vi "identify objects.vi"(0 "location":cluster{"x":i16, "y":i16}, 1 "8-bit pixmap":u8[][](array[numeric]), 3 "index":u8, 4 "navigational matrix":T1(array[cluster])) -> (5 "direction":dbl[](array[numeric]), 6 "distance":u16[](array[numeric]))   [LabVIEW 2009]
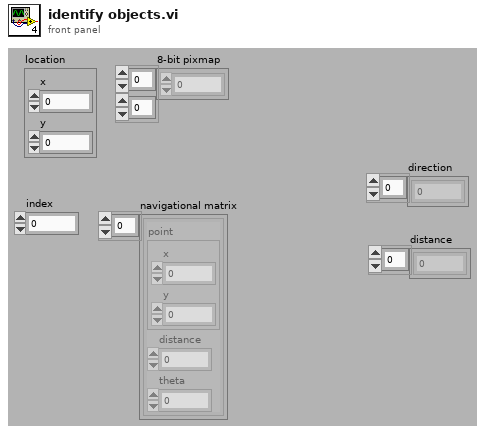
[diagram p1: front panel]
types:
  T1 = cluster{"point":cluster{"x":i16, "y":i16}, "distance":u16, "theta":dbl}[]
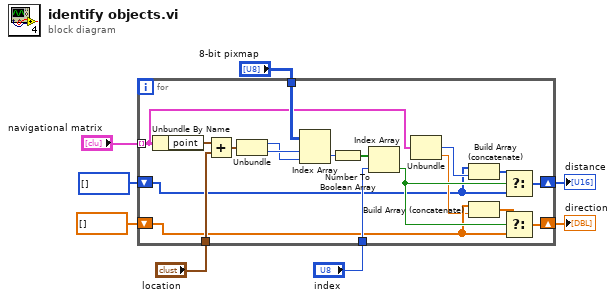
[diagram p0: block diagram]
diagram:
  n1 = for {
    tunnel: "navigational matrix" -> [w17] mode=indexing
    tunnel: "location" -> [w27]
    tunnel: "8-bit pixmap" -> [w23]
    tunnel: "index" -> [w20]
    shift-right: [w15] -> w1
    shift-left: dbl[] [] -> [w13]
    shift-right: [w16] -> w2
    shift-left: u16[] [] -> [w9]
    n2 = Unbundle By Name(w17) -> ("point"=w19:cluster{"x":i16, "y":i16})
    n3 = Add(x=w19, y=w27) -> (x+y=w26:cluster{"x":i16, "y":i16})
    n4 = Unbundle(w26) -> ("x"=w24:i16, "y"=w25:i16)
    n5 = Index Array(array=w23, index (row)=w25, index (col)=w24) -> (element=w22:u8)
    n6 = Number To Boolean Array(number=w22) -> (Boolean array=w21:bool[])
    n7 = Index Array(array=w21, index=w20) -> (element=w18:bool)
    n8 = Unbundle(w17) -> ("distance"=w10:u16, "theta"=w11:dbl)  [unwired: 1 out]
    n9 = Build Array (concatenate)(w9, w10) -> (w12:u16[])
    n10 = Build Array (concatenate)(w13, w11) -> (w14:dbl[])
    n11 = Select(t=w12, s=w18, f=w9) -> (s? t:f=w16:u16[])
    n12 = Select(t=w14, s=w18, f=w13) -> (s? t:f=w15:dbl[])
  }
  "distance" <- w2
  "direction" <- w1
